vi "Update display current.vi"(8 "error in (no error)":errorcluster, 11 "StageSPIM in":refnum<class "StageSPIM.lvclass">) -> (0 "error out":errorcluster, 3 "StageSPIM out":refnum<class "StageSPIM.lvclass">)   [LabVIEW 2012, in "StageSPIM.lvclass"]
uses:
  StageSPIM.lvclass
  StageSPIM.lvclass/StageSPIM.ctl
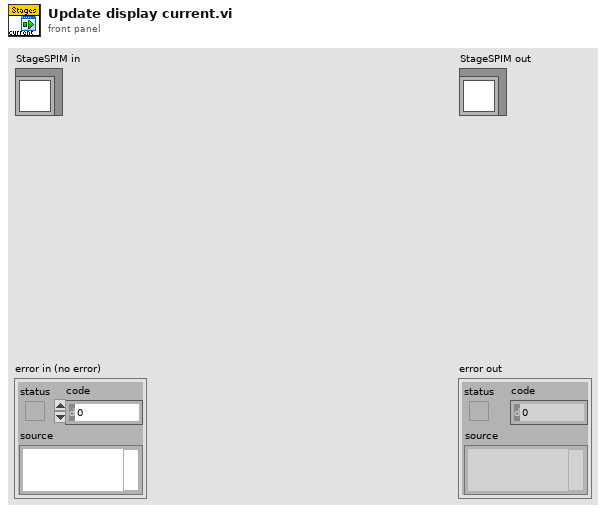
[diagram p1: front panel]
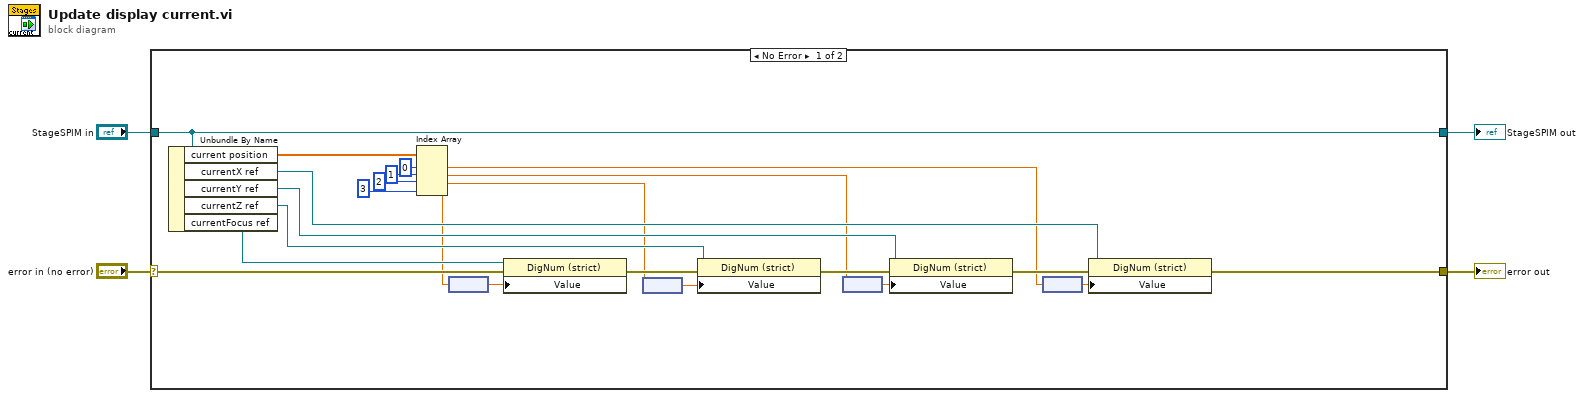
[diagram p0: block diagram]
diagram:
  n1 = case shown="No Error" "error in (no error)" {
    selector: "error in (no error)" -> [w12 w29]
    tunnel: [w9 w29] -> w3
    tunnel: [w27 w28] -> w1
    tunnel: "StageSPIM in" -> [w27 w28]
    frame No Error {
      n2 = Unbundle By Name(w27) -> ("current position"=w26:dbl[], "currentX ref"=w19:refnum<vi>, "currentY ref"=w20:refnum<vi>, "currentZ ref"=w21:refnum<vi>, "currentFocus ref"=w10:refnum<vi>)
      n3 = Index Array(array=w26, index #1=0 ("index"), index #2=1 ("index"), index #3=2 ("index"), index #4=3 ("index")) -> (element #1=w8:dbl, element #2=w7:dbl, element #3=w6:dbl, element #4=w5:dbl)
      n4 = node(w5) -> (w13:dbl[unit])
      n5 = property class="DigNum (strict)"(reference=w10, error in=w12, "Value"=w13) -> (error out=w11:errorcluster)  [unwired: 1 out]
      n6 = node(w6) -> (w16:dbl[unit])
      n7 = property class="DigNum (strict)"(reference=w21, error in=w11, "Value"=w16) -> (error out=w18:errorcluster)  [unwired: 1 out]
      n8 = node(w7) -> (w15:dbl[unit])
      n9 = property class="DigNum (strict)"(reference=w20, error in=w18, "Value"=w15) -> (error out=w17:errorcluster)  [unwired: 1 out]
      n10 = node(w8) -> (w14:dbl[unit])
      n11 = property class="DigNum (strict)"(reference=w19, error in=w17, "Value"=w14) -> (error out=w9:errorcluster)  [unwired: 1 out]
    }
    frame Error {
    }
  }
  "error out" <- w3
  "StageSPIM out" <- w1
